vi "HEWH Convert Cluster to String Test Profiles.vi"(8 "error in (no error)":errorcluster, 11 "24HR Test - High Usage Example":T1[](array[typedef]) {"Time" format="%<%H:%M:%S>t"}) -> (0 "error out":errorcluster, 3 "String Conversion":string[][](array[string]))   [LabVIEW 2020]
uses:
  Type Definitions/PRAT Test.ctl
  Utility/Save File/File Setup (Public)/Type Definition/Save File HEWH Heating Control Mode.ctl
  Draw Water Specific/Type Definitions/Terminate Draw Conditions.ctl
  Type Definitions/HEWH Start Conditions.ctl
  Draw Water Specific/Type Definitions/Check Special Condtions.ctl
  Draw Water Specific/Type Definitions/HEWH Special Condition Check.ctl
  Type Definitions/HEWH Draw Flag ENUM.ctl
  Utility/Save File/File Setup.lvlib
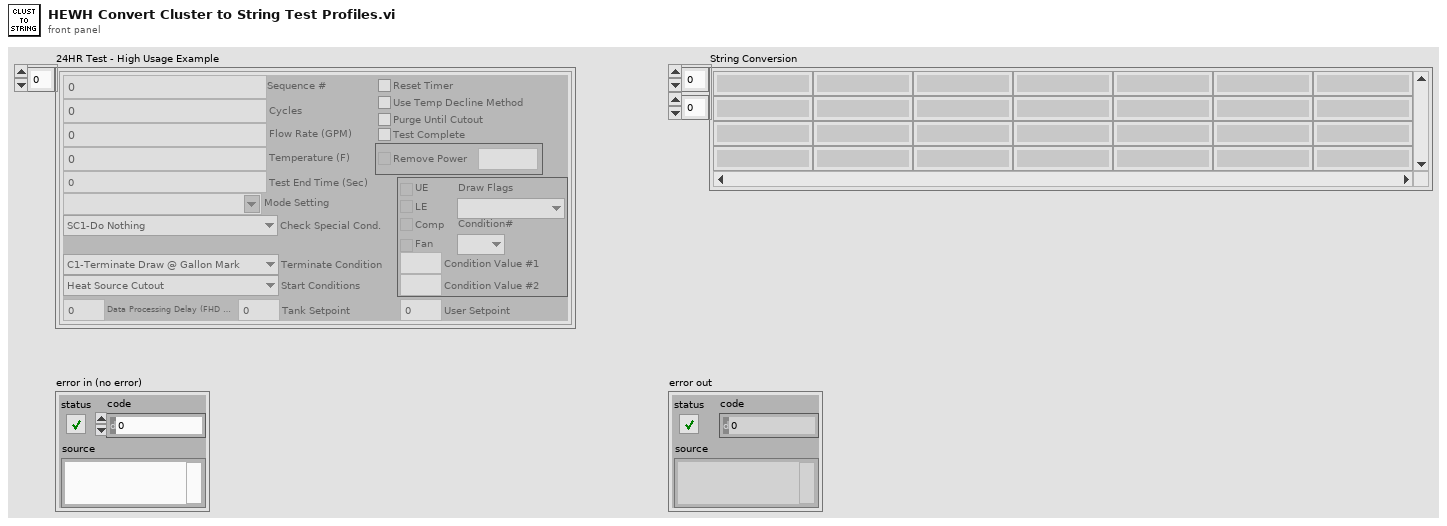
[diagram p1: front panel]
types:
  T1 = typedef "PRAT Test.ctl" = cluster{"Sequence #":dbl, "Cycles":i32, "Mode Setting":T2, "Flow Rate (GPM)":dbl, "Temperature (F)":dbl, "Reset Timer":bool, "Use Temp Decline Method":bool, "Terminate Condition":T3, "Condition Value #1":dbl, "UE":bool, "LE":bool, "Comp":bool, "Fan":bool, "Test End Time (Sec)":dbl, "Purge Until Cutout":bool, "Start Conditions":T4, "Condition Value #2":dbl, "Remove Power":bool, "Time":dbl, "Check Special Cond.":T5, "Condition#":T6, "Draw Flags":T7, "Data Processing Delay (FHD 15sec, UEF 5 Sec)":dbl, "Test Complete":bool, "User Setpoint":dbl, "Tank Setpoint":dbl}
  T2 = typedef "File Setup.lvlib/Save File HEWH Heating Control Mode.ctl" = string
  T3 = typedef "Terminate Draw Conditions.ctl" = enum16{"C1-Terminate Draw @ Gallon Mark", "C2-Special Last Draw (HU Test)", "C3-RTD Out <=", "C4-Mean Tank Temp <=", "C5-Decrease RTD Out (Deg F)", "C6-Time (Seconds)", "C7-Until Any Heat Source", "C8-Specific Heat Source", "C9-Do Nothing", "C10-Inlet Outlet RTD Temp Delta"}
  T4 = typedef "HEWH Start Conditions.ctl" = enum16{"Heat Source Cutout", "At Time (Seconds)", "Every X (Seconds)", "T2 >= X° Below Setpoint", "Seconds From Complete", "Wait for LE & Comp Cutout", "Wait for Comp Cutout", "Wait for LE Cutout", "Wait for UE Cutout", "Start Immediately"}
  T5 = typedef "Check Special Condtions.ctl" = enum16{"SC1-Do Nothing", "SC2-Check Heat Source (On-C2/Off-C1)", "SC3-Check Skip Condition", "SC4-Check Heat Source ON/Fail", "SC5-Keep Draw Valves Open", "SC6-Skip Purge"}
  T6 = typedef "HEWH Special Condition Check.ctl" = enum16{"N/A", "C1", "C2", "Reset/Fail", "Skip Draw Sequence"}
  T7 = typedef "HEWH Draw Flag ENUM.ctl" = enum16{"N/A", "None(0)", "Sml(1)", "Med(2)", "SmlMed(3)", "Lrg(4)", "SmlLrg(5)", "MedLrg(6)", "SmlMedLrg(7)"}
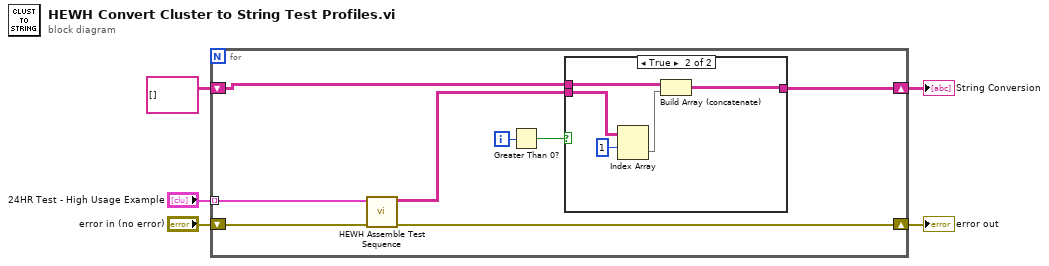
[diagram p0: block diagram]
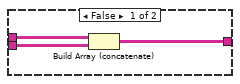
[diagram p2: hidden frame]
diagram:
  n1 = for {
    tunnel: "24HR Test - High Usage Example" -> [w13] mode=indexing
    shift-right: [w6] -> w3
    shift-left: string[][] [] -> [w12]
    shift-right: [w10] -> w2
    shift-left: "error in (no error)" -> [w9]
    i -> [w8]
    n2 = call "HEWH Assemble Test Sequence.vi"("Error In"=w9, "Cluster"=w13) -> ("Error Out"=w10:errorcluster, "String Test Seq"=w11:string[][])  [unwired: 8 in]
    n3 = Greater Than 0?(x=w8) -> (x > 0?=w7:bool)
    n4 = case shown="True" w7 {
      tunnel: w12 -> [w16 w21]
      tunnel: w11 -> [w15 w20]
      tunnel: [w14 w17] -> w6
      frame False {
        n5 = Build Array (concatenate)(w16, w15) -> (w14:string[][])
      }
      frame True {
        n6 = Index Array(array=w20, index (row)=1) -> (element=w18:string[])  [unwired: 1 in]
        n7 = Build Array (concatenate)(w21, w18) -> (w17:string[][])
      }
    }
  }
  "String Conversion" <- w3
  "error out" <- w2
